vi "Lim_FileGetImageRectData.vi"(8 "error in (no error)":errorcluster, 9 "frameindex":u32, 10 "LIMATTRIBUTES":T1, 11 "hFile in":T3) -> (0 "error out":errorcluster, 1 "LIMLOCALMETADATA":T2 {"dTimeMSec" format="%.2f"}, 3 "hFile out":T3)   [LabVIEW 2014, in "ND2_Reader_32.lvlib"]
uses:
  ND2_Reader_32.lvlib
  controls/numeric_LIMFILEHANDLE.ctl
  controls/numeric_LIMRESULT.ctl
  controls/cluster_LIMLOCALMETADATA.ctl
  controls/cluster_LIMATTRIBUTES.ctl
  nd2 reader/SDK/bin/x86/v6_w32_nd2ReadSDK.dll
panel:
  out "pBuffer":u8[](array[numeric])
  out "LIMRESULT":T4 items=["LIM_OK"=0, "LIM_ERR_UNEXPECTED"=-1, "LIM_ERR_NOTIMPL"=-2, "LIM_ERR_OUTOFMEMORY"=-3, "LIM_ERR_INVALIDARG "=-4, "LIM_ERR_NOINTERFACE"=-5, "LIM_ERR_POINTER"=-6, "LIM_ERR_FAIL"=-9, "LIM_ERR_NOTFOUND"=-13]
  # "This Routine does not work in LabVIEW"
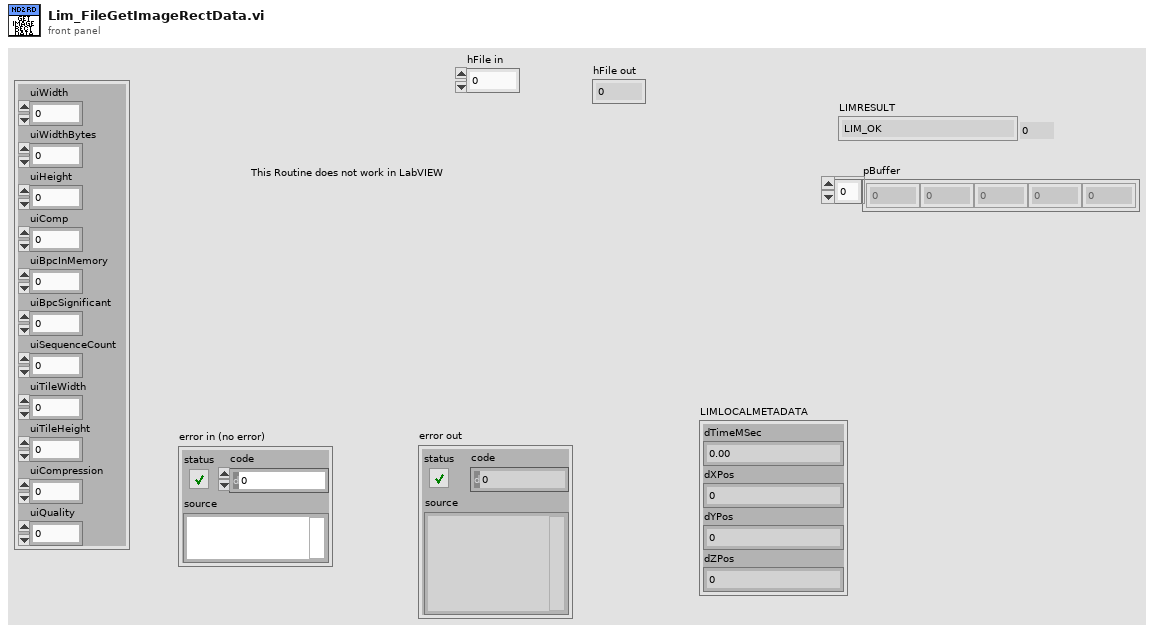
[diagram p1: front panel]
types:
  T1 = typedef "cluster_LIMATTRIBUTES.ctl" = cluster{"uiWidth":u32, "uiWidthBytes":u32, "uiHeight":u32, "uiComp":u32, "uiBpcInMemory":u32, "uiBpcSignificant":u32, "uiSequenceCount":u32, "uiTileWidth":u32, "uiTileHeight":u32, "uiCompression":u32, "uiQuality":u16}
  T2 = typedef "cluster_LIMLOCALMETADATA.ctl" = cluster{"dTimeMSec":dbl, "dXPos":dbl, "dYPos":dbl, "dZPos":dbl}
  T3 = typedef "numeric_LIMFILEHANDLE.ctl" = i32
  T4 = typedef "numeric_LIMRESULT.ctl" = i32
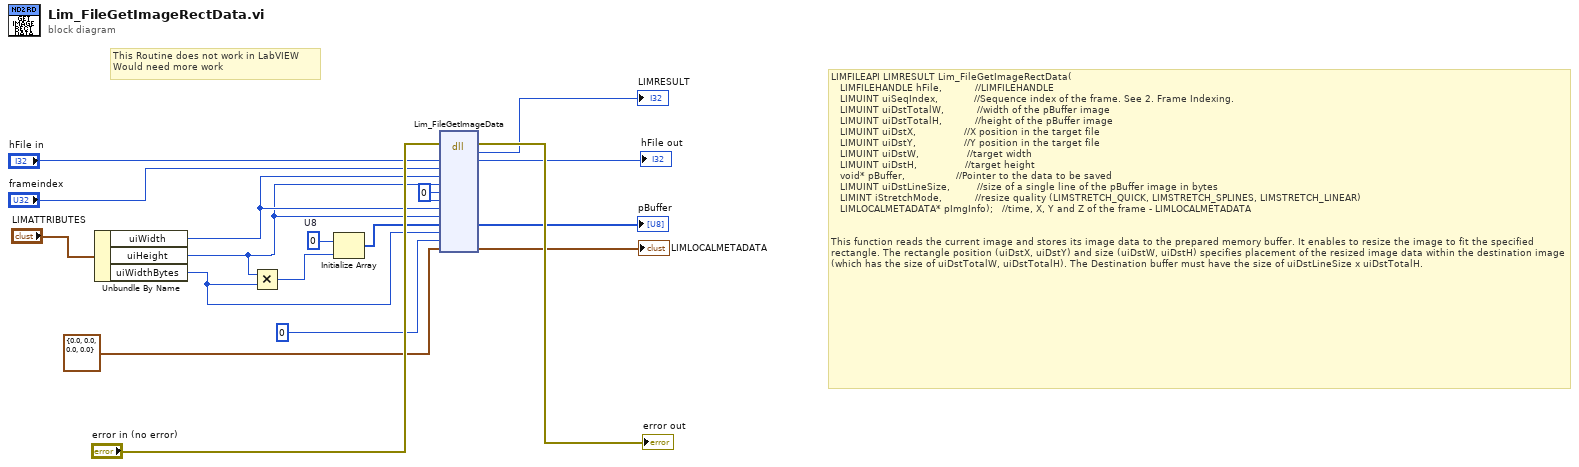
[diagram p0: block diagram]
diagram:
  w8 = u8 0  # U8
  w10 = u32 0 ("uiDstX")
  # "This Routine does not work in LabVIEW\nWould need more work"
  # "LIMFILEAPI LIMRESULT Lim_FileGetImageRectData(\n   LIMFILEHANDLE hFile,           //LIMFILEHANDLE \n   LIMUINT uiSeqIndex,            //Sequence index of the frame. See 2. Frame Indexing.\n   LIMUINT uiDstTotalW,           //width of the pBuffer image\n   LIMUINT uiDstTotalH,           //height of the pBuffer image\n   LIMUINT uiDstX,                //X position in the target file\n   LIMUINT uiDstY,                //Y position in the target file\n   LIMUINT uiDstW,                //target width\n   LIMUINT uiDstH,                //target height\n   void* pBuffer,                 //Pointer to the data to be saved\n   LIMUINT uiDstLineSize,         //size of a single line of the pBuffer image in bytes\n   LIMINT iStretchMode,           //resize quality (LIMSTRETCH_QUICK, LIMSTRETCH_SPLINES, LIMSTRETCH_LINEAR) \n   LIMLOCALMETADATA* pImgInfo);   //time, X, Y and Z of the frame - LIMLOCALMETADATA \n\n         \nThis function reads the current image and stores its image data to the prepared memory buffer. It enables to resize the image to fit the specified rectangle. The rectangle position (uiDstX, uiDstY) and size (uiDstW, uiDstH) specifies placement of the resized image data within the destination image (which has the size of uiDstTotalW, uiDstTotalH). The Destination buffer must have the size of uiDstLineSize x uiDstTotalH."
  n1 = Unbundle By Name("LIMATTRIBUTES") -> ("uiWidth"=w6:u32, "uiHeight"=w3:u32, "uiWidthBytes"=w4:u32)
  n2 = Multiply(x=w3, y=w4) -> (x*y=w2:u32)
  n3 = Initialize Array(w8, w2) -> (w5:u8[])
  n4 = dll-call lib="C:/Users/VirtualUser/Desktop/EPA-Vision/EPA Image Source LV2014 2.0.0 2016-02-23/ND2_Reader_32bit/nd2 reader/SDK/bin/x86/v6_w32_nd2ReadSDK.dll" fn="Lim_FileGetImageData"(error in="error in (no error)", "hFile"="hFile in", "uiSeqIndex"="frameindex", "uiDstTotalW"=w6, "uiDstTotalH"=w3, "uiDstX"=w10, "uiDstY"=w10, "uiDstW"=w6, "uiDstH"=w3, "pBuffer"=w5, "uiDstLineSize"=w4, "iStretchMode"=u32 0, "pImgInfo"=T2 {"dTimeMSec"=0.0, "dXPos"=0.0, "dYPos"=0.0, "dZPos"=0.0} ("LIMLOCALMETADATA")) -> (error out=→"error out":errorcluster, "LIMRESULT"=→"LIMRESULT":i32, "hFile"=→"hFile out":i32, "pBuffer"=→"pBuffer":u8[], "pImgInfo"=→"LIMLOCALMETADATA":T2)  [unwired: 2 in, 10 out]
